vi "ADI_IMU_ADIS16448_Open.vi"(8 "error in":errorcluster, 9 "AHRS Algorithm":enum16{"Complementary", "Madgwick"}(ring), 10 "Yaw Axis":enum16{"X", "Y", "Z"}(ring)=enum."Z", 11 "SPI Chip Select":T3=enum."SPI MXP") -> (0 "error out":errorcluster, 3 "ADI IMU Interrupt DevRef":T1={"ADI IMU DevRef"={"DevStatus"={"status"=FALSE, "code"=0, "source"=""}, "Handle"=0, "SPI Bus"=enum."SPI On-Board, CS0", "Device Found"=FALSE, "Device Ready"=FALSE, "Yaw Axis"=enum."Z", "AHRS Algorithm"=enum."Complementary", "Serial"=0, "Lot ID 2"=0, "Lot ID 1"=0, "Product ID"=0}, "InterruptRef"={"DevStatus"={"status"=FALSE, "code"=0, "source"=""}, "InterruptIndex"=enum."0"}})   [LabVIEW 2016, in "ADIS16448_IMU.lvlib"]
doc: "Initiates communication between an Analog Devices MXP IMU and the RoboRIO."
uses:
  ADIS16448_IMU.lvlib
  <vilib>/Rock Robotics/SystemInterfaces/spilib/spi_bus.ctl
  ADI_IMU_ADIS16448_InterruptDevRef.ctl
  ADI_IMU_ADIS16448_IMUDevRef.ctl
  <vilib>/Rock Robotics/WPI/Interrupt/WPI_InterruptRef.ctl
  <vilib>/Rock Robotics/SystemInterfaces/Interrupt/FPGA_InterruptIndex.ctl
  <vilib>/Rock Robotics/WPI/SPI/WPI_SPIMode.ctl
  <vilib>/Rock Robotics/SystemInterfaces/DIO/FPGA_DIOChannel.ctl
  <vilib>/Rock Robotics/SystemInterfaces/NetworkCommunication/NetComm_UsageReport_ResourceType.ctl
  ADI_IMU_ADIS16448_Registers.ctl
  <vilib>/Rock Robotics/WPI/Counter/WPI_CounterDigitalInputToDigitalSource.vi
  <vilib>/Rock Robotics/SystemInterfaces/CounterEncoderSourceConvertion/FPGA_CounterEncoderSourceConvertionLVSourceTypeToFPGAType.vi
  <vilib>/Rock Robotics/WPI/Interrupt/WPI_InterruptCache.vi
  <vilib>/Rock Robotics/SystemInterfaces/Interrupt/FPGA_InterruptWriteConfiguration.vi
  ADI_IMU_ADIS16448_Loop.vi
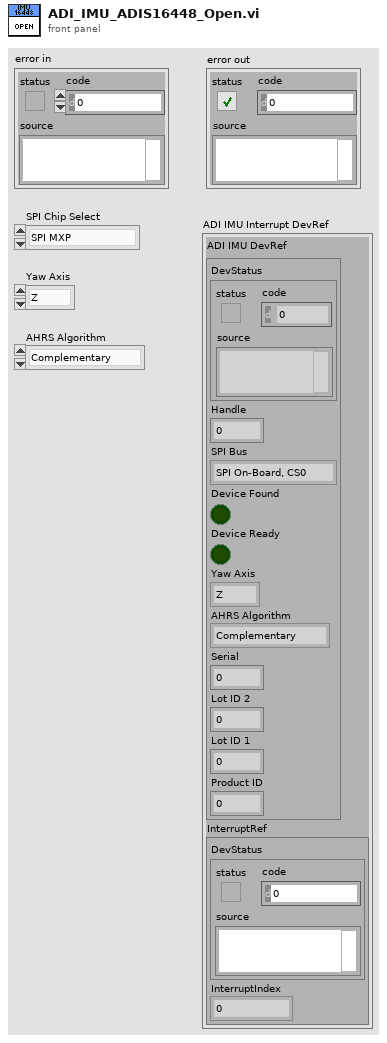
[diagram p1: front panel]
types:
  T1 = typedef "ADIS16448_IMU.lvlib/ADI_IMU_ADIS16448_InterruptDevRef.ctl" = cluster{"ADI IMU DevRef":T2, "InterruptRef":T4}
  T2 = typedef "ADIS16448_IMU.lvlib/ADI_IMU_ADIS16448_IMUDevRef.ctl" = cluster{"DevStatus":errorcluster, "Handle":i32, "SPI Bus":T3, "Device Found":bool, "Device Ready":bool, "Yaw Axis":enum16{"X", "Y", "Z"}, "AHRS Algorithm":enum16{"Complementary", "Madgwick"}, "Serial":u16, "Lot ID 2":u16, "Lot ID 1":u16, "Product ID":u16}
  T3 = typedef "spi_bus.ctl" = enum16{"SPI On-Board, CS0", "SPI On-Board, CS1", "SPI On-Board, CS2", "SPI On-Board, CS3", "SPI MXP", "Invalid"}
  T4 = typedef "WPI_InterruptRef.ctl" = cluster{"DevStatus":errorcluster, "InterruptIndex":T5}
  T5 = typedef "FPGA_InterruptIndex.ctl" = enum8{"0", "1", "2", "3", "4", "5", "6", "7", "Invalid"}
  T6 = typedef "NetComm_UsageReport_ResourceType.ctl" = enum8{"Controller", "Module", "Language", "CANPlugin", "Accelerometer", "ADXL345", "AnalogChannel", "AnalogTrigger", "AnalogTriggerOutput", "CANJaguar", "Compressor", "Counter", "Dashboard", "DigitalInput", "DigitalOutput", "DriverStationCIO", "DriverStationEIO", "DriverStationLCD", "Encoder", "GearTooth", "Gyro", "I2C", "Framework", "Jaguar", "Joystick", "Kinect", "KinectStick", "PIDController", "Preferences", "PWM", "Relay", "RobotDrive", "SerialPort", "Servo", "Solenoid", "SPI", "Task", "Ultrasonic", "Victor", "Button", "Command", "AxisCamera", "PCVideoServer", "SmartDashboard", "Talon", "HiTechnicColorSensor", "HiTechnicAccel", "HiTechnicCompass", "SRF08", "AnalogOutput", "Victor SP", "Talon SRX", "CAN Talon SRX", "ADXL362 Accel", "ADXRS450 Gyro", "Rev SPARK", "Mindsensors SD540", "Digital Filter", "ADIS16448", "PDP", "PCM", "PigeonIMU"}
  T7 = typedef "FPGA_DIOChannel.ctl" = enum8{"DIO 0", "DIO 1", "DIO 2", "DIO 3", "DIO 4", "DIO 5", "DIO 6", "DIO 7", "DIO 8", "DIO 9", "DIO MXP 0", "DIO MXP 1", "DIO MXP 2", "DIO MXP 3", "DIO MXP 4", "DIO MXP 5", "DIO MXP 6", "DIO MXP 7", "DIO MXP 8", "DIO MXP 9", "DIO MXP 10", "DIO MXP 11", "DIO MXP 12", "DIO MXP 13", "DIO MXP 14", "DIO MXP 15", "SPI Port CS1", "SPI Port CS2", "SPI Port CS3", "SPI Port MISO", "SPI Port MOSI", "Invalid"}
  T8 = typedef "WPI_SPIMode.ctl" = enum16{"Mode 0 (Clk Idle Low,Sample on Leading)", "Mode 1 (Clk Idle Low,Sample on Trailing)", "Mode 2 (Clk Idle High,Sample on Leading)", "Mode 3 (Clk Idle High,Sample on Trailing)"}
  T9 = typedef "ADIS16448_IMU.lvlib/ADI_IMU_ADIS16448_Registers.ctl" = u8
  T10 = typedef "WPI_DigitalOutputDevRef.ctl" = cluster{"DIO Channel":T7, "DevStatus":errorcluster}
  T11 = typedef "WPI_DigitalInputDevRef.ctl" = cluster{"DevStatus":errorcluster, "DIO Channel":T7}
  T12 = typedef "WPI_SPIDevRef.ctl" = cluster{"DevStatus":errorcluster, "Handle":i32, "SPI Bus":T3}
  T13 = typedef "FPGA_CounterEncoderSourceConvertionLVSourceType.ctl" = cluster{"DevStatus":errorcluster, "AnalogTriggerMode?":bool, "DigitalMode":cluster{"DIO Channel":T14}, "AnalogTriggerMode":cluster{"AnalogTriggerIndex":T15, "OutputType":T16}}
  T14 = typedef "FPGA_DIODigitalSourceChannel.ctl" = enum8{"DIO 0", "DIO 1", "DIO 2", "DIO 3", "DIO 4", "DIO 5", "DIO 6", "DIO 7", "DIO 8", "DIO 9", "DIO MXP 0", "DIO MXP 1", "DIO MXP 2", "DIO MXP 3", "DIO MXP 4", "DIO MXP 5", "DIO MXP 6", "DIO MXP 7", "DIO MXP 8", "DIO MXP 9", "DIO MXP 10", "DIO MXP 11", "DIO MXP 12", "DIO MXP 13", "DIO MXP 14", "DIO MXP 15", "Disabled"}
  T15 = typedef "FPGA_AnalogTriggerIndex.ctl" = enum8{"Trig 0", "Trig 1", "Trig 2", "Trig 3", "Trig 4", "Trig 5", "Trig 6", "Trig 7", "Invalid"}
  T16 = typedef "FPGA_AnalogTriggerOutType.ctl" = enum16{"InWindow", "TriggerState", "Rising", "Falling"}
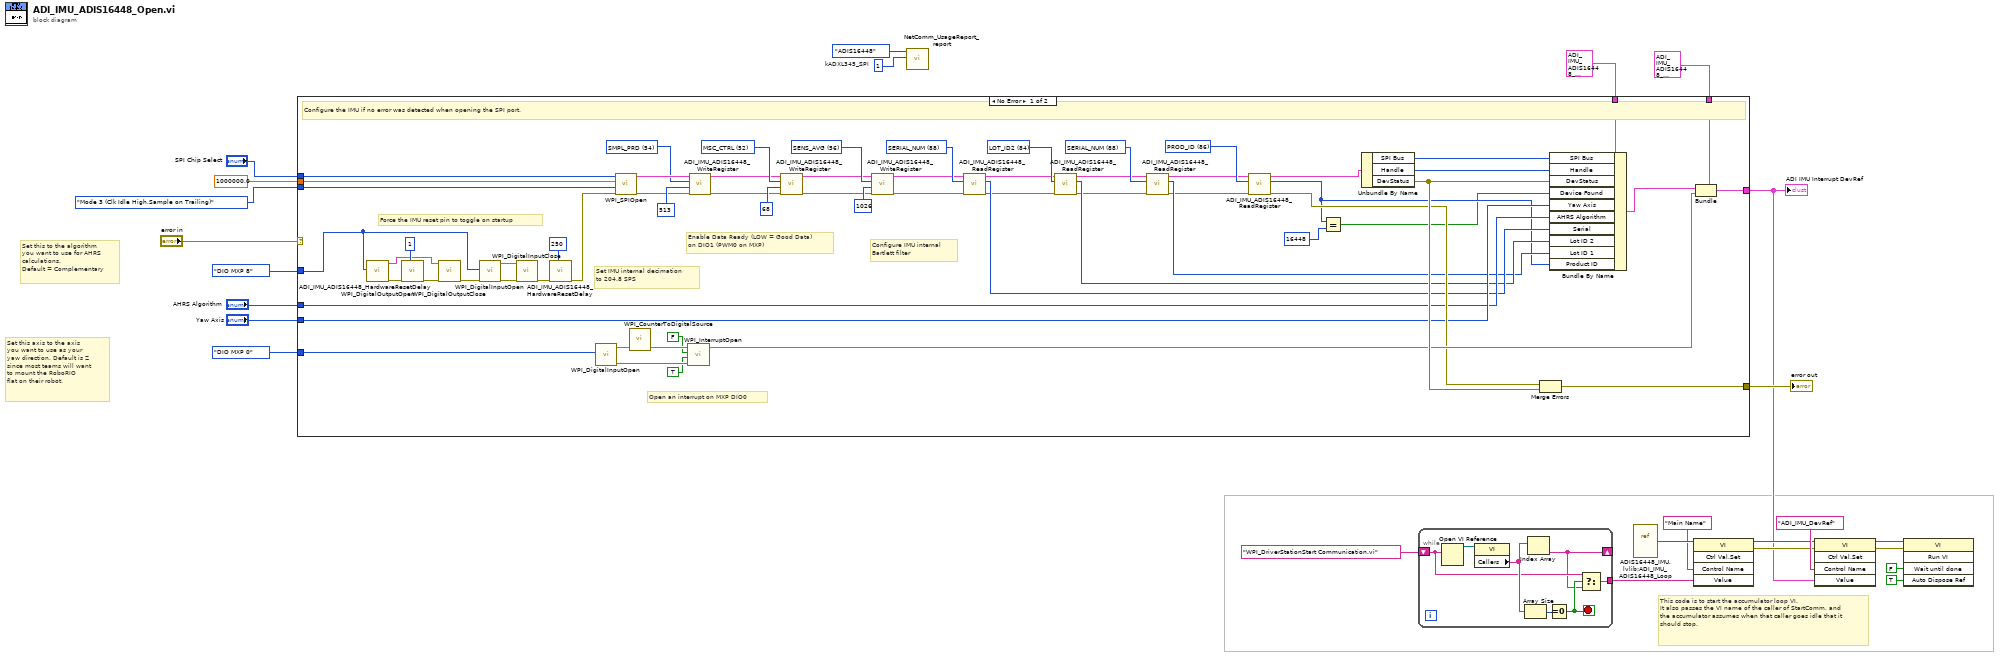
[diagram p0: block diagram]
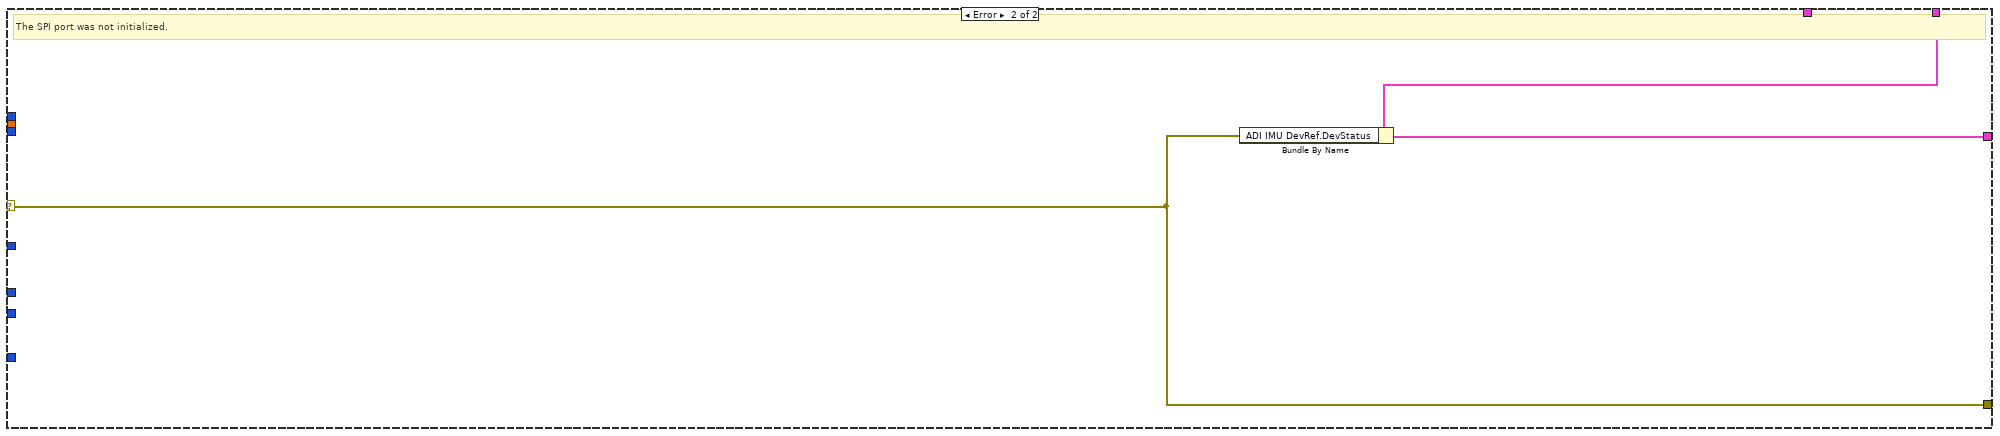
[diagram p2: hidden frame]
diagram:
  w14 = u8 1  # kADXL345_SPI
  # "This code is to start the accumulator loop VI.\nIt also passes the VI name of the caller of StartComm, and the accumulator assumes when that caller goes idle that it should stop."
  # "Set this to the algorithm\nyou want to use for AHRS\ncalculations. \nDefault = Complementary"
  # "Set this axis to the axis\nyou want to use as your\nyaw direction. Default is Z\nsince most teams will want \nto mount the RoboRIO\nflat on their robot."
  n1 = case shown="No Error" "error in" {
    selector: "error in" -> [_ w90]
    tunnel: "SPI Chip Select" -> [w88 _]
    tunnel: 1000000.0 ("Clock Rate (Hz)") -> [w87 _]
    tunnel: WPI_SPIMode."Mode 3 (Clk Idle High,Sample on Trailing)" ("Mode (3)") -> [w86 _]
    tunnel: [w80 w90] -> w21
    tunnel: T2 {"DevStatus"={"status"=FALSE, "code"=0, "source"=""}, "Handle"=0, "SPI Bus"=enum."SPI On-Board, CS0", "Device Found"=FALSE, "Device Ready"=FALSE, "Yaw Axis"=enum."Z", "AHRS Algorithm"=enum."Complementary", "Serial"=0, "Lot ID 2"=0, "Lot ID 1"=0, "Product ID"=0} ("SimpleGyroDevRef 2") -> [w85 _]
    tunnel: [w71 w89] -> w1
    tunnel: T1 {"ADI IMU DevRef"={"DevStatus"={"status"=FALSE, "code"=0, "source"=""}, "Handle"=0, "SPI Bus"=enum."SPI On-Board, CS0", "Device Found"=FALSE, "Device Ready"=FALSE, "Yaw Axis"=enum."Z", "AHRS Algorithm"=enum."Complementary", "Serial"=0, "Lot ID 2"=0, "Lot ID 1"=0, "Product ID"=0}, "InterruptRef"={"DevStatus"={"status"=FALSE, "code"=0, "source"=""}, "InterruptIndex"=enum."0"}} ("output cluster") -> [w70 w91]
    tunnel: FPGA_DIOChannel."DIO MXP 0" ("DIO Channel") -> [w69 _]
    tunnel: "Yaw Axis" -> [w64 _]
    tunnel: "AHRS Algorithm" -> [w63 _]
    tunnel: FPGA_DIOChannel."DIO MXP 8" ("DIO Channel") -> [w28 _]
    frame No Error {
      w45 = T9 86 items=["GLOB_CMD"=62, "SEQ_CNT"=58, "SMPL_PRD"=54, "SENS_AVG"=56, "MSC_CTRL"=52, "ERROR_FLAGS"=60, "TEMP"=44, "BARO"=40, "Z_MAG"=36, "Y_MAG"=32, "X_MAG"=28, "Z_ACCEL"=24, "Y_ACCEL"=20, "X_ACCEL"=16, "Z_GYRO"=12, "Y_GYRO"=8, "X_GYRO"=4, "PROD_ID"=86, "LOT_ID2"=84, "LOT_ID1"=82, "SERIAL_NUM"=88] ("ADIS16448 Register")
      w46 = T9 88 items=["GLOB_CMD"=62, "SEQ_CNT"=58, "SMPL_PRD"=54, "SENS_AVG"=56, "MSC_CTRL"=52, "ERROR_FLAGS"=60, "TEMP"=44, "BARO"=40, "Z_MAG"=36, "Y_MAG"=32, "X_MAG"=28, "Z_ACCEL"=24, "Y_ACCEL"=20, "X_ACCEL"=16, "Z_GYRO"=12, "Y_GYRO"=8, "X_GYRO"=4, "PROD_ID"=86, "LOT_ID2"=84, "LOT_ID1"=82, "SERIAL_NUM"=88] ("ADIS16448 Register")
      w48 = T9 84 items=["GLOB_CMD"=62, "SEQ_CNT"=58, "SMPL_PRD"=54, "SENS_AVG"=56, "MSC_CTRL"=52, "ERROR_FLAGS"=60, "TEMP"=44, "BARO"=40, "Z_MAG"=36, "Y_MAG"=32, "X_MAG"=28, "Z_ACCEL"=24, "Y_ACCEL"=20, "X_ACCEL"=16, "Z_GYRO"=12, "Y_GYRO"=8, "X_GYRO"=4, "PROD_ID"=86, "LOT_ID2"=84, "LOT_ID1"=82, "SERIAL_NUM"=88] ("ADIS16448 Register")
      w51 = T9 88 items=["GLOB_CMD"=62, "SEQ_CNT"=58, "SMPL_PRD"=54, "SENS_AVG"=56, "MSC_CTRL"=52, "ERROR_FLAGS"=60, "TEMP"=44, "BARO"=40, "Z_MAG"=36, "Y_MAG"=32, "X_MAG"=28, "Z_ACCEL"=24, "Y_ACCEL"=20, "X_ACCEL"=16, "Z_GYRO"=12, "Y_GYRO"=8, "X_GYRO"=4, "PROD_ID"=86, "LOT_ID2"=84, "LOT_ID1"=82, "SERIAL_NUM"=88] ("ADIS16448 Register")
      w52 = T9 56 items=["GLOB_CMD"=62, "SEQ_CNT"=58, "SMPL_PRD"=54, "SENS_AVG"=56, "MSC_CTRL"=52, "ERROR_FLAGS"=60, "TEMP"=44, "BARO"=40, "Z_MAG"=36, "Y_MAG"=32, "X_MAG"=28, "Z_ACCEL"=24, "Y_ACCEL"=20, "X_ACCEL"=16, "Z_GYRO"=12, "Y_GYRO"=8, "X_GYRO"=4, "PROD_ID"=86, "LOT_ID2"=84, "LOT_ID1"=82, "SERIAL_NUM"=88] ("ADIS16448 Register")
      w53 = T9 52 items=["GLOB_CMD"=62, "SEQ_CNT"=58, "SMPL_PRD"=54, "SENS_AVG"=56, "MSC_CTRL"=52, "ERROR_FLAGS"=60, "TEMP"=44, "BARO"=40, "Z_MAG"=36, "Y_MAG"=32, "X_MAG"=28, "Z_ACCEL"=24, "Y_ACCEL"=20, "X_ACCEL"=16, "Z_GYRO"=12, "Y_GYRO"=8, "X_GYRO"=4, "PROD_ID"=86, "LOT_ID2"=84, "LOT_ID1"=82, "SERIAL_NUM"=88] ("ADIS16448 Register")
      w54 = T9 54 items=["GLOB_CMD"=62, "SEQ_CNT"=58, "SMPL_PRD"=54, "SENS_AVG"=56, "MSC_CTRL"=52, "ERROR_FLAGS"=60, "TEMP"=44, "BARO"=40, "Z_MAG"=36, "Y_MAG"=32, "X_MAG"=28, "Z_ACCEL"=24, "Y_ACCEL"=20, "X_ACCEL"=16, "Z_GYRO"=12, "Y_GYRO"=8, "X_GYRO"=4, "PROD_ID"=86, "LOT_ID2"=84, "LOT_ID1"=82, "SERIAL_NUM"=88] ("ADIS16448 Register")
      # "Force the IMU reset pin to toggle on startup"
      # "Open an interrupt on MXP DIO0"
      # "Configure IMU internal\nBartlett filter"
      # "Enable Data Ready (LOW = Good Data) \non DIO1 (PWM0 on MXP)"
      # "Set IMU internal decimation\nto 204.8 SPS"
      # "Configure the IMU if no error was detected when opening the SPI port."
      n2 = call <vilib>:"WPI_DigitalOutputOpen.vi"("DIO Channel"=w28) -> ("error out"=w58:errorcluster, "DigitalOutputDevRef"=w26:T10)  [unwired: 9 in]
      n3 = call "ADI_IMU_ADIS16448_HardwareResetDelay.vi"("Delay (ms)"=u32 1, "error in"=w58) -> ("error out"=w59:errorcluster)  [unwired: 9 in]
      n4 = call <vilib>:"WPI_DigitalOutputClose.vi"("error in (no error)"=w59, "DigitalOutputDevRef"=w26) -> ("error out"=w57:errorcluster)  [unwired: 9 in]
      n5 = call <vilib>:"WPI_DigitalInputOpen.vi"("error in (no error)"=w57, "DIO Channel"=w28) -> ("error out"=w56:errorcluster, "DigitalInputDevRef"=w55:T11)  [unwired: 8 in]
      n6 = call <vilib>:"WPI_DigitalInputClose.vi"("error in (no error)"=w56, "DigitalInputDevRef"=w55) -> ("error out"=w43:errorcluster)  [unwired: 9 in]
      n7 = call "ADI_IMU_ADIS16448_HardwareResetDelay.vi"("Delay (ms)"=u32 250, "error in"=w43) -> ("error out"=w42:errorcluster)  [unwired: 9 in]
      n8 = call <vilib>:"WPI_DigitalInputOpen.vi"("DIO Channel"=w69) -> ("error out"=w76:errorcluster, "DigitalInputDevRef"=w78:T11)  [unwired: 9 in]
      n9 = call <vilib>:"WPI_SPIOpen.vi"("error in"=w42, "Mode (3)"=w86, "Clock Rate (Hz)"=w87, "SPI Bus"=w88) -> ("error out"=w60:errorcluster, "SPIDevRef"=w61:T12)  [unwired: 6 in]
      n10 = call-poly <vilib>:"WPI_CounterToDigitalSource.vi"("DigitalInputDevRef"=w78) -> ("Digital Source"=w77:T13)  [unwired: 6 in]
      n11 = call <vilib>:"WPI_InterruptOpen.vi"("error in (no error)"=w76, "Falling Edge"=TRUE, "Rising Edge"=FALSE, "Source"=w77) -> ("InterruptRef"=w73:T4)  [unwired: 6 in, 1 out]
      n12 = call "ADI_IMU_ADIS16448_WriteRegister.vi"("error in (no error)"=w60, "Data"=u16 513, "ADIS16448 Register"=w54, "SPIDevRef in"=w61) -> ("error out"=w39:errorcluster, "SPIDevRef out"=w40:T12)  [unwired: 6 in]
      n13 = call "ADI_IMU_ADIS16448_WriteRegister.vi"("error in (no error)"=w39, "Data"=u16 68, "ADIS16448 Register"=w53, "SPIDevRef in"=w40) -> ("error out"=w37:errorcluster, "SPIDevRef out"=w38:T12)  [unwired: 6 in]
      n14 = call "ADI_IMU_ADIS16448_WriteRegister.vi"("error in (no error)"=w37, "Data"=u16 1026, "ADIS16448 Register"=w52, "SPIDevRef in"=w38) -> ("error out"=w35:errorcluster, "SPIDevRef out"=w36:T12)  [unwired: 6 in]
      n15 = call "ADI_IMU_ADIS16448_ReadRegister.vi"("error in (no error)"=w35, "ADIS16448 Register"=w51, "SPIDevRef in"=w36) -> ("error out"=w33:errorcluster, "Register Value"=w50:u16, "SPIDevRef out"=w34:T12)  [unwired: 6 in]
      n16 = call "ADI_IMU_ADIS16448_ReadRegister.vi"("error in (no error)"=w33, "ADIS16448 Register"=w48, "SPIDevRef in"=w34) -> ("error out"=w31:errorcluster, "Register Value"=w49:u16, "SPIDevRef out"=w32:T12)  [unwired: 6 in]
      n17 = call "ADI_IMU_ADIS16448_ReadRegister.vi"("error in (no error)"=w31, "ADIS16448 Register"=w46, "SPIDevRef in"=w32) -> ("error out"=w29:errorcluster, "Register Value"=w47:u16, "SPIDevRef out"=w30:T12)  [unwired: 6 in]
      n18 = call "ADI_IMU_ADIS16448_ReadRegister.vi"("error in (no error)"=w29, "ADIS16448 Register"=w45, "SPIDevRef in"=w30) -> ("error out"=w67:errorcluster, "Register Value"=w44:u16, "SPIDevRef out"=w68:T12)  [unwired: 6 in]
      n19 = Equal?(x=w44, y=u16 16448) -> (x = y?=w27:bool)
      n20 = Unbundle By Name(w68) -> ("SPI Bus"=w84:T3, "Handle"=w83:i32, "DevStatus"=w81:errorcluster)
      n21 = Merge Errors(w67, w81) -> (w80:errorcluster)
      n22 = Bundle By Name(cluster=w85, "SPI Bus"=w84, "Handle"=w83, "DevStatus"=w81, "Device Found"=w27, "Yaw Axis"=w64, "AHRS Algorithm"=w63, "Serial"=w50, "Lot ID 2"=w49, "Lot ID 1"=w47, "Product ID"=w44) -> (w72:T2)
      n23 = Bundle(cluster=w70, "ADI IMU DevRef"=w72, "InterruptRef"=w73) -> (w71:T1)
    }
    frame Error {
      # "The SPI port was not initialized."
      n24 = Bundle By Name(cluster=w91, "ADI IMU DevRef.DevStatus"=w90) -> (w89:T1)
    }
  }
  "error out" <- w21
  "ADI IMU Interrupt DevRef" <- w1
  n25 = call <vilib>:"NetComm_UsageReport_report.vi"("Instance Number"=w14, "Resource Type"=NetComm_UsageReport_ResourceType."ADIS16448") -> ()  [unwired: 10 in]
  n26 = while {
    shift-right: [w93] -> _
    shift-left: "WPI_DriverStationStart Communication.vi" -> [w94]
    tunnel: [w92] -> w3
    stop <- w95 stop-if-true
    n27 = Open VI Reference(vi path=w94) -> (vi reference=w98:refnum<vi>)  [unwired: 1 in, 5 out]
    n28 = property class="VI"(reference=w98) -> ("Callers"=w96:string[])  [unwired: 1 in, 2 out]
    n29 = Array Size(array=w96) -> (size(s)=w97:i32)
    n30 = Index Array(array=w96) -> (element=w93:string)  [unwired: 1 in]
    n31 = Equal To 0?(x=w97) -> (x = 0?=w95:bool)
    n32 = Select(t=w94, s=w95, f=w93) -> (s? t:f=w92:string)
  }
  n33 = vi-ref "ADIS16448_IMU.lvlib:ADI_IMU_ADIS16448_Loop.vi"() -> (w5:refnum<vi>)
  n34 = invoke class="VI" method="Ctrl Val.Set"(reference=w5, "Control Name"="Main Name", "Value"=w3) -> (reference out=w2:refnum<vi>, error out=w7:errorcluster)  [unwired: 2 in, 3 out]
  n35 = invoke class="VI" method="Ctrl Val.Set"(reference=w2, error in=w7, "Control Name"="ADI_IMU_DevRef", "Value"=w1) -> (reference out=w12:refnum<vi>, error out=w8:errorcluster)  [unwired: 1 in, 3 out]
  n36 = invoke class="VI" method="Run VI"(reference=w12, error in=w8, "Wait until done"=FALSE ("Wait Until Done"), "Auto Dispose Ref"=TRUE ("Auto Dispose Reference")) -> ()  [unwired: 1 in, 5 out]
